vi "Read Last Series Index.vi"(11 "Results in":refnum<class "Results.lvclass">) -> (2 "Series index":i32, 3 "Results out":refnum<class "Results.lvclass">)   [LabVIEW 2018, in "InfluxDB Client.lvlib" / "Results.lvclass"]
uses:
  Results.lvclass
  Results.lvclass/Results.ctl
  Result/Result.lvclass/Result.ctl
  Result/Result.lvclass
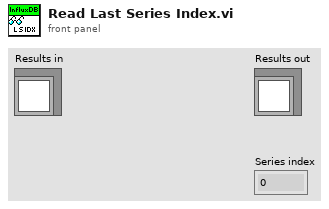
[diagram p1: front panel]
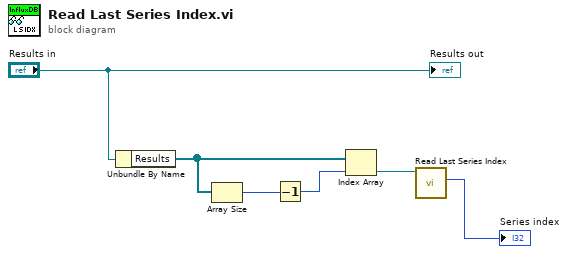
[diagram p0: block diagram]
diagram:
  n1 = Unbundle By Name("Results in") -> ("Results"=w4:refnum<class "Result.lvclass">[])
  n2 = Array Size(array=w4) -> (size(s)=w5:i32)
  n3 = Decrement(x=w5) -> (x-1=w3:i32)
  n4 = Index Array(array=w4, index=w3) -> (element=w2:refnum<class "Result.lvclass">)
  n5 = call "Read Last Series Index.vi"("Result in"=w2) -> ("Series Index"=→"Series index":i32)  [unwired: 9 in, 1 out]
  "Results out" <- "Results in"
